vi "Math Marker Data.vi"(8 "error in (no error)":errorcluster, 9 "Marker Function (0: Flatness)":u16(ring) items=["Flatness", "RF Filter Statistics", "Statistics"], 10 "Channel (1)":i32=1, 11 "VISA resource name":refnum<visa-resource-name>) -> (0 "error out":errorcluster, 1 "Num3":dbl, 2 "Num2":dbl, 3 "VISA resource name out":refnum<visa-resource-name>, 4 "Num4":dbl, 5 "Num1":dbl)   [LabVIEW 2012, in "Tektronix TTR500 Series.lvlib"]
doc: "For the active trace of channel, returns marker flatness or filter statistics or marker statistics data."
uses:
  <instrlib>/Tektronix TTR500 Series/Tektronix TTR500 Series.lvlib
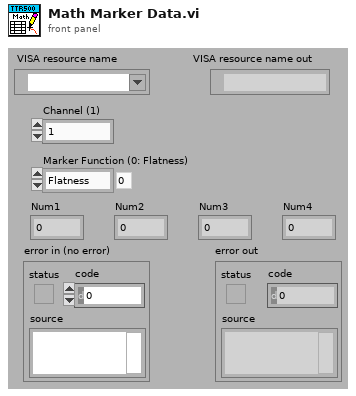
[diagram p1: front panel]
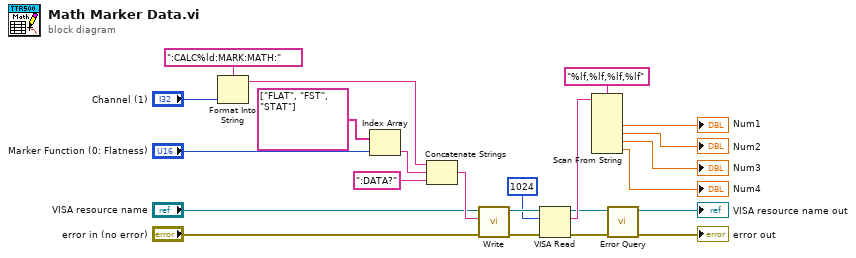
[diagram p0: block diagram]
diagram:
  n1 = Format Into String(format string=":CALC%ld:MARK:MATH:", "Channel (1)") -> (resulting string=w5:string)  [unwired: 2 in, 1 out]
  n2 = Index Array(array=string[] ["FLAT", "FST", "STAT"], index="Marker Function (0: Flatness)") -> (element=w6:string)
  n3 = Concatenate Strings(w5, w6, ":DATA?") -> (w15:string)
  n4 = call <instrlib>:"Write.vi"("error in (no error)"="error in (no error)", "String ()"=w15, "VISA resource name"="VISA resource name") -> ("error out"=w13:errorcluster, "VISA resource name out"=w14:refnum<visa-resource-name>)  [unwired: 6 in, 1 out]
  n5 = VISA Read(VISA resource name=w14, byte count=u32 1024, error in (no error)=w13) -> (VISA resource name out=w4:refnum<visa-resource-name>, read buffer=w11:string, error out=w3:errorcluster)  [unwired: 1 out]
  n6 = Scan From String(format string="%lf,%lf,%lf,%lf", input string=w11) -> (output 1=→"Num1":dbl, output 2=→"Num2":dbl, output 3=→"Num3":dbl, output 4=→"Num4":dbl)  [unwired: 6 in, 3 out]
  n7 = call <instrlib>:"Error Query.vi"("error in (no error)"=w3, "VISA resource name"=w4) -> ("error out"=→"error out":errorcluster, "VISA resource name out"=→"VISA resource name out":refnum<visa-resource-name>)  [unwired: 6 in, 2 out]
